vi "AlliGator Add Phasor Value to Plot v2.vi"(0 "Phasor Graph Ref":refnum<vi>, 1 "Calibration Phasor":T12, 5 "Phasor Data in":T2 {"[Phasor Graph:Raw Phasor Plots]"."[Decay Metadata]"."# Folds" min=1; "[Phasor Graph:Raw Phasor Plots]"."[Decay Metadata]"."ROI Descriptor"."Contours"."Type" items=["No Selection", "Point", "Line", "Rectangle", "Oval", "Polygon", "Freehand Region", "Annulus", "Unused2", "Unused3", "Broken Line", "Freehand Line", "Rotated Rectangle"]}, 7 "Decay":cluster{"t Array":dbl[], "I Array":dbl[]}, 9 "ROI Decay  Metadata":T4={"ROI Descriptor"={"Global Rectangle"=[], "Contours"=[]}, "ROI Center"={"X"=0, "Y"=0}, "Decay Background Subtraction Info"={"Laser Period"=0.0, "Gate Duration"=0.0, "Baseline Subtraction Method"=enum."Mean", "Background Definition Range"={"Min Gate"=0.0, "Max Gate"=0.0}, "Total Intensity w/o Bkgd Subtraction"=0.0, "Bkgd-subtracted Intensity (exp)"=0.0, "# Data Points"=0, "Background/Gate"=0.0, "Fitted Lifetime"=0.0, "Bkgd-subtracted Intensity (theo)"=0.0}, "Decay Reverted"=FALSE, "Decay Smoothened"=FALSE, "Decay Straightened"=FALSE, "Fitted Tau (Decay Straightening)"=0.0, "Decay Shift Parameters"={"Type"=enum."Default", "Shift"=0.0, "Threshold"=0.0, "Rotate"=FALSE}, "Decay Shifted"=FALSE, "Decay Extrapolated"=FALSE, "Decay Extrapolation Parameters"={"Additional Points"=0, "Head Fraction"=0.0, "Fitted Tau"=0.0, "Use Periodicity"=FALSE, "Use Cursors"=FALSE, "Tail Fraction"=0.0}, "Decay Normalized"=FALSE, "Fold Decay"=FALSE, "# Folds"=1} {"# Folds" min=1; "ROI Descriptor"."Contours"."Type" items=["No Selection", "Point", "Line", "Rectangle", "Oval", "Polygon", "Freehand Region", "Annulus", "Unused2", "Unused3", "Broken Line", "Freehand Line", "Rotated Rectangle"]}, 11 "Error In":errorcluster, 12 "Single Step Phasor":refnum<vi>) -> (2 "Raw Phasor":T1, 3 "Calibrated Phasor":T1, 4 "Phasor Data out":T2 {"[Phasor Graph:Raw Phasor Plots]"."[Decay Metadata]"."# Folds" min=1; "[Phasor Graph:Raw Phasor Plots]"."[Decay Metadata]"."ROI Descriptor"."Contours"."Type" items=["No Selection", "Point", "Line", "Rectangle", "Oval", "Polygon", "Freehand Region", "Annulus", "Unused2", "Unused3", "Broken Line", "Freehand Line", "Rotated Rectangle"]}, 8 "Raw Phasor SDV":T1, 10 "Calibrated Phasor SDV":T1, 13 "Apparent Phase Lifetime":dbl[unit], 14 "Message":string, 15 "Error Out":errorcluster)   [LabVIEW 2021, in "AlliGator Phasor Graph.lvlib"]
doc: "Core VI handling the creation of a phasor plot in the Phasor Graph.\n\nFrom the <B>Decay</B> plot and <B>Calibration Phasor</b>, computes the phasor (and if selected, the phasor standard deviation due to shot noise) and adds it to the current Phasor Plot in the Phasor Graph."
uses:
  AlliGator Phasor Graph.lvlib
  Phasor/Phasor (g, s).ctl
  Phasor/Calibration Phasor (m, phi).ctl
  AlliGator Decay Metadata v3.ctl
  Decay Analysis/Decay Preprocessing/AlliGator Decay Background Subtraction Info.ctl
  Decay Analysis/Decay Preprocessing/AlliGator Baseline Subtraction Method.ctl
  Graphs/XY Graph/XY Graph Plot Shift Parameters.ctl
  Graphs/XY Graph/XY Graph Plot Shift Method.ctl
  Decay Analysis/Decay Preprocessing/AlliGator Decay Extrapolation Parameters.ctl
  AlliGator Phasor Data.ctl
  AlliGator Raw Phasor Plot Data v4.ctl
  Phasor/Phasor Standard Deviation Options.ctl
  Settings/AlliGator Settings List.ctl
  Globals, Variables, Constants/AlliGator Variables List.ctl
  AlliGator Raw Phasor Plot Array Action.ctl
  dd0b4273-0e3d-468f-9a24-7a5fea4f6c4e.vi
  Variant/Variant to Data/Variant to Boolean.vi
  Phasor/Phasor.lvlib
  Settings/AlliGator Settings.lvlib
  Graphs/XY Graph/XY Graph Add-Ons.lvlib
  Error/Error.lvlib
  Phasor Ratio/AlliGator Phasor Ratio.lvlib
  Globals, Variables, Constants/AlliGator Globals, Variables & Constants.lvlib
  Variant/Variant to Data/Variant to Data.lvlib
  Decay Analysis/Decay Preprocessing/AlliGator Decay Preprocessing.lvlib
panel:
  # "see the AlliGator License on the block diagram (Ctrl+E or Window:Show Block Diagram)"
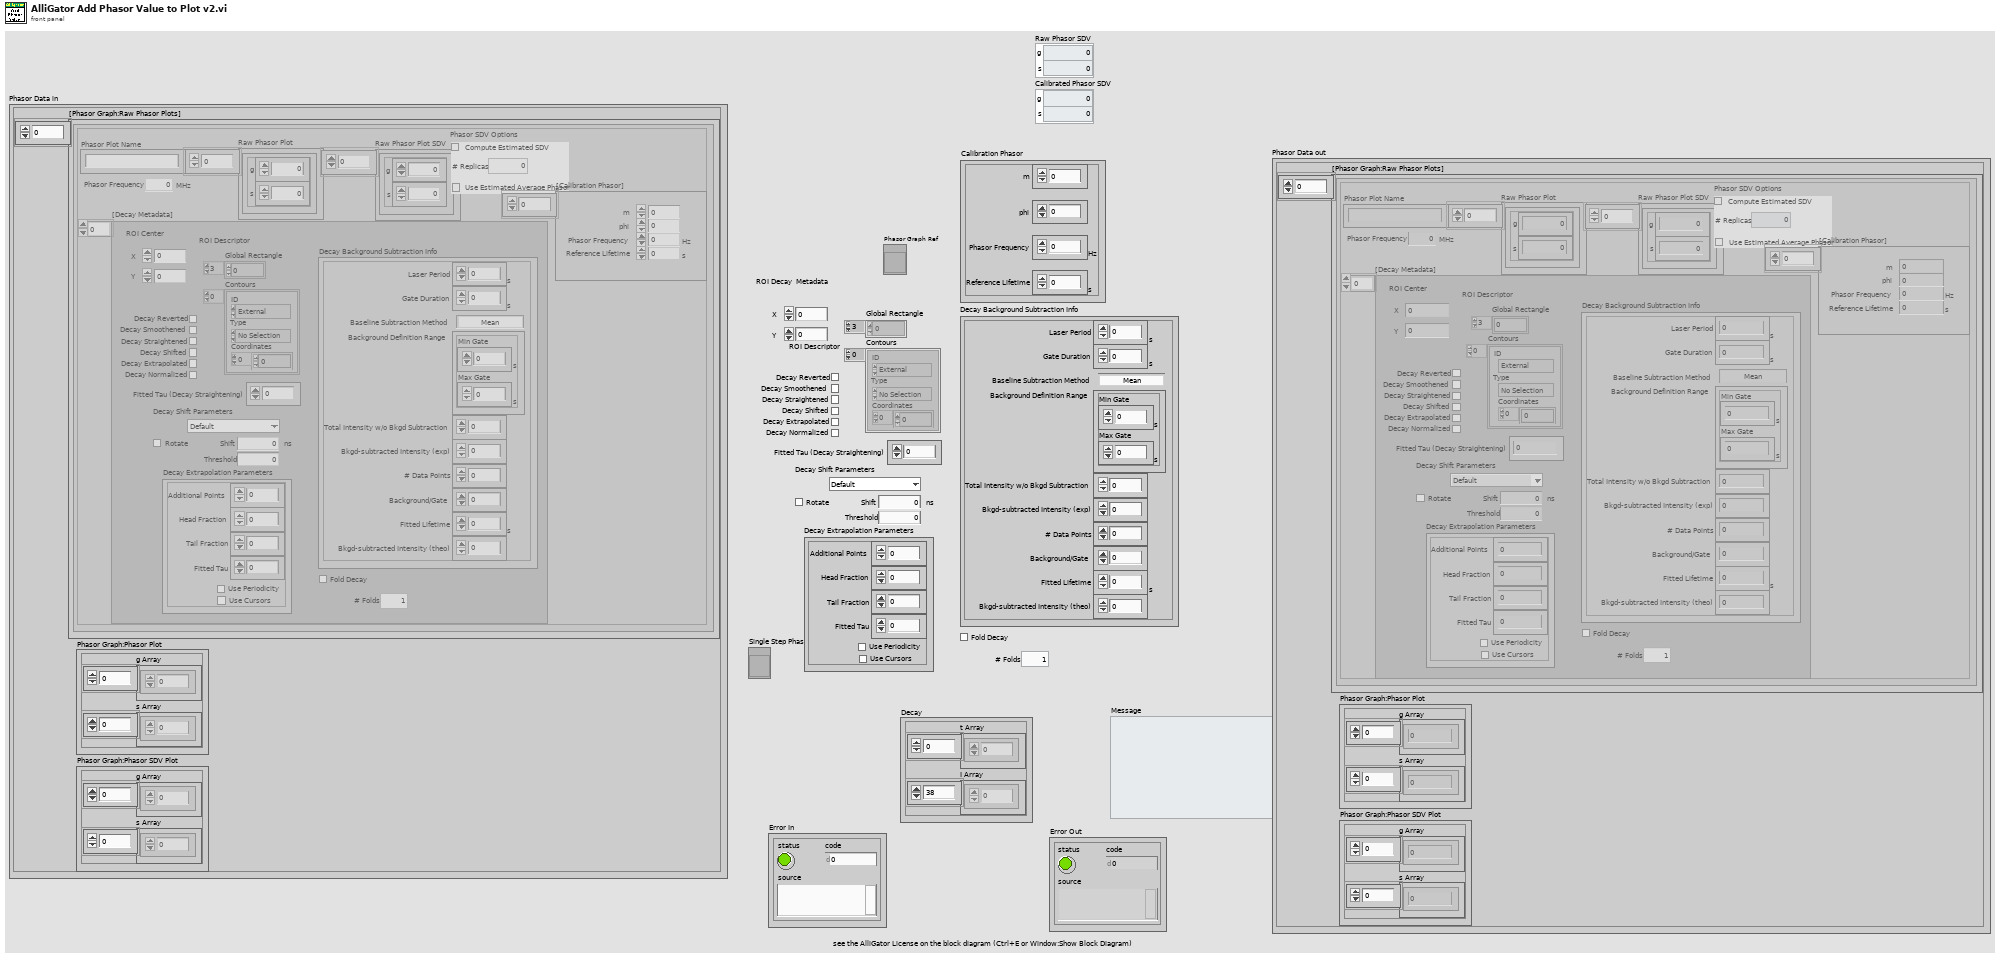
[diagram p1: front panel]
types:
  T1 = typedef "Phasor.lvlib/Phasor (g, s).ctl" = cluster{"g":dbl, "s":dbl}
  T2 = typedef "AlliGator Phasor Graph.lvlib/AlliGator Phasor Data.ctl" = cluster{"[Phasor Graph:Raw Phasor Plots]":T3[], "Phasor Graph:Phasor Plot":cluster{"g Array":dbl[], "s Array":dbl[]}, "Phasor Graph:Phasor SDV Plot":cluster{"g Array":dbl[], "s Array":dbl[]}}
  T3 = typedef "AlliGator Phasor Graph.lvlib/AlliGator Raw Phasor Plot Data v4.ctl" = cluster{"Phasor Plot Name":string, "Raw Phasor Plot":T1[], "Phasor Frequency":dbl[unit], "[Decay Metadata]":T4[], "Raw Phasor Plot SDV":T1[], "Phasor SDV Options":T11, "[Calibration Phasor]":T12[]}
  T4 = typedef "AlliGator Phasor Graph.lvlib/AlliGator Decay Metadata v3.ctl" = cluster{"ROI Descriptor":T5, "ROI Center":cluster{"X":i32, "Y":i32}, "Decay Background Subtraction Info":T6, "Decay Reverted":bool, "Decay Smoothened":bool, "Decay Straightened":bool, "Fitted Tau (Decay Straightening)":dbl, "Decay Shift Parameters":T8, "Decay Shifted":bool, "Decay Extrapolated":bool, "Decay Extrapolation Parameters":T10, "Decay Normalized":bool, "Fold Decay":bool, "# Folds":u32}
  T5 = typedef "ROI Descriptor" = cluster{"Global Rectangle":i32[], "Contours":cluster{"ID":enum32{"External", "Internal"}, "Type":u32, "Coordinates":i32[]}[]}
  T6 = typedef "AlliGator Decay Preprocessing.lvlib/AlliGator Decay Background Subtraction Info.ctl" = cluster{"Laser Period":dbl[unit], "Gate Duration":dbl[unit], "Baseline Subtraction Method":T7, "Background Definition Range":cluster{"Min Gate":dbl[unit], "Max Gate":dbl[unit]}, "Total Intensity w/o Bkgd Subtraction":dbl, "Bkgd-subtracted Intensity (exp)":dbl, "# Data Points":i32, "Background/Gate":dbl, "Fitted Lifetime":dbl[unit], "Bkgd-subtracted Intensity (theo)":dbl}
  T7 = typedef "AlliGator Decay Preprocessing.lvlib/AlliGator Baseline Subtraction Method.ctl" = enum16{"Mean", "Min", "Square Gated Single-Exponential", "File", "Constant"}
  T8 = typedef "XY Graph Add-Ons.lvlib/XY Graph Plot Shift Parameters.ctl" = cluster{"Type":T9, "Shift":dbl[unit], "Threshold":dbl, "Rotate":bool}
  T9 = typedef "XY Graph Add-Ons.lvlib/XY Graph Plot Shift Method.ctl" = enum16{"Default", "CFD", "Threshold", "Cross-Correlation"}
  T10 = typedef "AlliGator Decay Preprocessing.lvlib/AlliGator Decay Extrapolation Parameters.ctl" = cluster{"Additional Points":u32, "Head Fraction":dbl, "Fitted Tau":dbl, "Use Periodicity":bool, "Use Cursors":bool, "Tail Fraction":dbl}
  T11 = typedef "Phasor.lvlib/Phasor Standard Deviation Options.ctl" = cluster{"Compute Estimated SDV":bool, "# Replicas":u32, "Use Estimated Average Phasor":bool}
  T12 = typedef "Phasor.lvlib/Calibration Phasor (m, phi).ctl" = cluster{"m":dbl, "phi":dbl, "Phasor Frequency":dbl[unit], "Reference Lifetime":dbl[unit]}
  T13 = typedef "AlliGator Settings.lvlib/AlliGator Settings List.ctl" = enum16{"GUI:Visible Settings Tab", "GUI:Last Run Version", "Source Image:Use Image Histogram for Contrast", "Source Image:Low Count Pixels Rejection Options", "Source Image:High Count Pixels Rejection Options", "Source Image:Use Image Brightness", "Source Image:Blend Overlay with Image Background", "Source Image:Use Fixed ROI Diameter", "Source Image:ROI Diameter", "Source Image:ROI Center Color", "Source Image:Peak Threshold", "Source Image:Intensity Threshold", "Source Image:Image Binning Options", "Source Image:Image Smoothing Options", "Source Image:Image Histogram Active", "Source Image:Invert Binary Mask", "Source Image:Hot Pixel Removal", "Source Image:Overlay Analyzed ROI Center", "Source Image:Auto-Adjust Contrast", "Source Image:Histogram Lower Percentile", "Source Image:Histogram Upper Percentile", "Source Image:Save Source Image", "Source Image:Scale Bar Options", "Source Image:Image Resolution (Pixel Size)", "Source Image:Flatfield Correction", "Source Image:Show Dead Left Columns Correction", "Source Image:Dead Left Columns Correction", "Source Image:Image Pre-Processing Operations Order", "Source Image:Overlay ROI Median", "Source Image:Median Overlay Color", "Data Information:Gate Width", "Data Information:Nanotime Gate Separation", "Data Information:Macrotime Gate Separation", "Data Information:Gate Step", "Data Information:# Gates", "Data Information:Gate Image Exposure", "Data Information:Gate Image Integration", "Data Information:Gates to Skip", "Data Information:Gates to Keep", "Data Information:Define Gates to", "Data Information:Channel Name", "Data Information:Available Channel Names", "Data Information:Channel Arithmetic", "Data Information:Background File Subtraction", "Data Information:Background File", "Data Information:Background Scaling Factor", "Data Information:Background Pile-up Correction", "Data Information:Background Pixel Well Capacity", "Data Information:Laser Period", "Data Information:SYNC Period", "Data Information:Pile-up Correction", "Data Information:Pixel Well Capacity", "Data Information:Dataset Scaling Factor", "Fluorescence Decay_Decay Pre-Processing:Reverse Gates", "Fluorescence Decay_Decay Pre-Processing:Verbose Decay Pre-Processing", "Fluorescence Decay_Decay Pre-Processing:Use Decay Pre-Processing", "Fluorescence Decay_Decay Pre-Processing:Background Subtraction", "Fluorescence Decay_Decay Pre-Processing:Background Definition Range", "Fluorescence Decay_Decay Pre-Processing:Baseline Subtraction Method", "Fluorescence Decay_Decay Pre-Processing:Decay Pre-Processing Operations Order", "Fluorescence Decay_Decay Pre-Processing:Smoothing Parameter", "Fluorescence Decay_Decay Pre-Processing:Shift Decay", "Fluorescence Decay_Decay Pre-Processing:Decay Shift Parameters", "Fluorescence Decay_Decay Pre-Processing:Fold Decay", "Fluorescence Decay_Decay Pre-Processing:# Folds", "Fluorescence Decay_Decay Pre-Processing:1-Normalize Decay", "Fluorescence Decay_Decay Pre-Processing:[0-1]-Normalize Decay", "Fluorescence Decay_Decay Pre-Processing:Smoothen Decay", "Fluorescence Decay_Decay Pre-Processing:Extrapolate Decay", "Fluorescence Decay_Decay Pre-Processing:Use Periodicity", "Fluorescence Decay_Decay Pre-Processing:Use Cursors", "Fluorescence Decay_Decay Pre-Processing:Tail Fraction", "Fluorescence Decay_Decay Pre-Processing:Head Fraction", "Fluorescence Decay_Decay Pre-Processing:Additional Points", "Fluorescence Decay_Decay Pre-Processing:Straighten Decay", "Fluorescence Decay_Decay Pre-Processing:Constant Background", "Fluorescence Decay_Decay Pre-Processing:Pixel-Normalize Decay", "Fluorescence Decay_Advanced Analysis:Extract IRF instead of Decay", "Fluorescence Decay_Advanced Analysis:IRF Extraction Options", "Fluorescence Decay_Advanced Analysis:IRF Optimization Options", "Fluorescence Decay_Advanced Analysis:Square Pulse Options", "Fluorescence Decay_Advanced Analysis:IRF Order", "Fluorescence Decay_Advanced Analysis:IRF Time Constants", "Fluorescence Decay_Advanced Analysis:Wavelet Analysis Options", "Fluorescence Decay_Advanced Analysis:Average Lifetime Options", "Fluorescence Decay_Fit Options:Fit Options", "Fluorescence Decay_Fit Options:Use Legacy Fitting Approach", "Fluorescence Decay_Fit Options:Use Data Information Laser Period", "Fluorescence Decay_Fit Parameters:Displayed Fit Parameters", "Fluorescence Decay_Fit Parameters:Fit Parameter Constraints", "Fluorescence Decay_Fit Parameters:Export Tabulated Results", "Fluorescence Decay_Fit Parameters:MLE Baseline Offset Type", "Fluorescence Decay_Fit Parameters:MLE Baseline Offset", "Fluorescence Decay_Fit Parameters:Guess Parameter Names", "Fluorescence Decay_Fit Parameters:Guess Parameter Values", "Fluorescence Decay_Fit Parameters:Guess Parameters Options", "Fluorescence Decay_Styles:Show Last Decay Only", "Fluorescence Decay_Styles:Decay Graph Color Array", "Fluorescence Decay:Decay Graph Active", "Fluorescence Decay Statistics:Min Peak Value", "Fluorescence Decay Statistics:Reject Low Decay Peak Pixels", "Fluorescence Decay Statistics:Reject High Decay Peak Pixels", "Fluorescence Decay Statistics:Max Peak Value", "Time Traces:Use File Timestamp", "Time Traces:Time Step", "Time Traces:Use Intensity Correction File", "Time Traces:Intensity Correction File", "Phasor Plot:Phasor Plot Smoothing Options", "Phasor Plot:Phasor Plot Size", "Phasor Plot:Phasor Plot Graphics Options", "Phasor Plot:Cumulative Phasor Plot", "Phasor Plot:Use Phasor Brightness", "Phasor Plot:Blend Overlay with Phasor Background", "Phasor Plot:Save Phasor Plot", "Phasor Plot:Show References", "Phasor Plot:Phasor Ratio Decay Range", "Phasor Plot:Exponential Fading", "Phasor Plot:Phasor Ratio Reference Colors", "Phasor Plot:Reference Radius", "Phasor Plot:Show Color Map Vertices", "Phasor Plot:Phasor Plot Active", "Phasor Plot:Phasor Ratio Color Map Type", "Phasor Plot:Phasor Ratio Color Map", "Phasor Plot:Phasor Ratio Display Range", "Phasor Plot:Selected Image ROI(s)", "Phasor Plot:All Image ROIs", "Phasor Plot:Selected Phasor Plot ROI(s)", "Phasor Plot:All Phasor Plot ROIs", "Phasor Plot:Phasor Ratio Color-Coded Quantity", "Phasor Plot:Store Phasor Harmonics", "Phasor Plot:Draw Reference Segment", "Phasor Plot:User-Defined Quantity", "Phasor Graph:Phasor Frequency", "Phasor Graph:Phasor Ratio Type", "Phasor Graph:Pixel-level Phasor Computation", "Phasor Graph:Save Phasor Graph", "Phasor Graph:Phasor Graph Active", "Phasor Graph:Phasor SDV Options", "Phasor Calibration:Use Backup Calibration if needed", "Phasor Graph:Define Shortest Lifetime as", "Phasor Calibration:Backup Calibration Type", "Phasor Calibration:Calibration Type", "Phasor Calibration:Calibration Lifetime", "Phasor Calibration:Calibration Map Algorithm", "Single-Exponential Phasor Locus (SEPL):Gate Parameters", "Single-Exponential Phasor Locus (SEPL):User-defined Gate", "Single-Exponential Phasor Locus (SEPL):User-defined IRF", "Single-Exponential Phasor Locus (SEPL):Phasor Parameters", "Single-Exponential Phasor Locus (SEPL):Decay & IRF Parameters", "Single-Exponential Phasor Locus (SEPL):Display Parameters", "Lifetime Analysis:Decay Analysis Parameters", "Lifetime Analysis:Lifetime Map Active", "Plugins:Python Settings", "Miscellaneous:Verbose Mode", "Miscellaneous:Beep after Script", "Miscellaneous:Saved Image File Format", "Miscellaneous:Exported Gate Image Settings", "Miscellaneous:Include Loading in Timing", "Miscellaneous:Verbose Settings Mode", "Miscellaneous:Histogram Options", "Miscellaneous:Beep on Error", "Miscellaneous:# Logical Processors Used", "Miscellaneous:ROI Description Max Characters", "Miscellaneous:Verbose Error Mode", "Miscellaneous:Transparent Mask Color"}
  T14 = typedef "AlliGator Globals, Variables & Constants.lvlib/AlliGator Variables List.ctl" = enum16{"---- GUI ----", "GUI:Initialization Status", "GUI:State Indicators Refnum", "GUI:Original AlliGator Menu Items", "GUI:Current Action Loop State", "GUI:Script in progress", "GUI:Playback", "GUI:Loop Playback", "GUI:Search ROI Used", "GUI:Search ROI", "Decay Graph Max Legend Size", "Intensity Graph Max Legend Size", "Decay Statistics Graph Max Legend Size", "Phasor Graph Max Legend Size", "Phasor Ratio Graph Max Legend Size", "Lifetime Graph Max Legend Size", "---- Files ----", "Files:Export Dataset Frames as Individual Files", "Files:Show Batch Export Help Balloons", "Files:Frames in Dataset", "Files:ptu File Frame Start Indices", "Files:Current Frame in Dataset", "Files:Current Frame Timestamp", "Files:Dataset Loaded", "Files:Dataset Metadata", "Files:Dataset Channel", "Files:Dataset Data Description", "Files:Background Dataset Metadata", "Files:Background Dataset Channel", "Files:Background Dataset Data Description", "Files:Background File Subtraction", "Files:Background File Path", "Files:Background File Pile-up Correction", "Files:Background File Pixel Well Capacity", "Files:Background File Scaling Factor", "Files:Current Dataset Load Settings", "Files:Dataset Path", "Files:ICCD-specific Information", "Files:Macrotime Gate Separation", "------ Python Plugins ------", "Python Plugins:Information", "Python Plugins:Python Session", "Python Plugins:Valid Python Session?", "---- Source Image ----", "Source Image:ROIs", "Source Image:Current ROI", "Source Image:ROI Event Refnum", "X_Source Image Display Range", "X_Source Image Palette Information", "X_Type of Displayed Image", "X_Time Gate Slider", "Source Image:Palette List", "Source Image:Scale", "Source Image:ROI Overlay Color", "Source Image:Overlay to Erase", "Source Image:Is Displayed Image Accumulated", "Source Image:White Light Image Modified", "Source Image:Mask Image Modified", "---- Image Profile Window ----", "Image Profile:Window Event Refnum", "Image Profile:IntensityType", "Image Profile:Intensity Average Type", "Image Profile:Intensity-weighted SDV", "Image Profile:Box Profile Type", "Image Profile:Window Open", "Image Profile:Plotted Fit Parameter", "------ Phasor Graph -------", "Phasor Graph:Show Line", "---- Phasor Plot ---", "Phasor Plot:Parameters Changed", "Phasor Plot:FLI Dataset Modified since last Calculation", "Phasor Harmonics Data", "Selected Phasor Harmonics", "Phasor Harmonic Manager Event Refnum", "Phasor Plot:ROIs", "Phasor Plot:Current ROI", "Phasor Plot:ROI Event Refnum", "Phasor Plot:Image Reference Points", "Phasor Plot:Computed", "Phasor Plot:Palette Information", "Phasor Plot:Palette List", "Phasor Plot:Phasor Ratio Palette Information", "Phasor Plot:Phasor Ratio Palette List", "Phasor Plot:Image Scale", "Phasor Plot:Image Overlay to Erase", "Phasor Plot:Image Elements to Update", "Phasor Plot:Current Calculation Parameters", "Phasor Plot:Current Calibration Options", "Phasor Plot:Reset Cumulated Phasor Plot", "Phasor Plot:Reference 1", "Phasor Plot:Lifetime Reference 1", "Phasor Plot:Reference 1 Frequency", "Phasor Plot:Reference 2", "Phasor Plot:Lifetime Reference 2", "Phasor Plot:Reference 2 Frequency", "---- Decay Analysis ----", "Number of Selected Decays to Fit", "LS Fit Results", "LAR Fit Results", "BS Fit Results", "Last Decay Max - Min", "Best Fit Parameters", "Best Fit Parameter Names", "Actual Size X", "Actual Size Y", "Binning X", "Binning Y", "Actual # Gates", "Dataset Number", "Gates to...", "Gates Skipped", "Gates to keep", "Gate Step", "Gate Separation", "Reversed Gates", "Pile-up Correction", "Pixel Well Capacity", "Background Subtracted", "Background Subtraction Method", "Background Definition Range", "Background File (deprecated)", "Number of Dataset Accumulated", "Array of Accumulated Dataset Paths", "Do Averaged Datasets", "Destination File Path", "Process Plot Target", "Use 1/D as Phasor Frequency", "---- Decay Fit Parameter Map -----", "Decay Fit Parameter Map:Palette Information", "Decay Fit Parameter Map:Palette List", "---- Parameter Map ----", "Parameter Map:Palette Information", "Parameter Map:Palette List", "------- Local Decay Window ---------", "Local Decay Graph Window:Event Refnum", "Local Decay Graph Window:Use normalized IRF for convolution", "----- Miscellaneous ----", "Misc:Skippable Dialog Windows Status"}
  T15 = typedef "AlliGator Phasor Graph.lvlib/AlliGator Raw Phasor Plot Array Action.ctl" = enum16{"Clear All", "-", "Add Raw Phasor Plot", "Delete Raw Phasor Plot", "Replace Raw Phasor Plot", "---------------------", "Add Phasor to Plot", "Replace Phasor in Plot", "Remove Phasor in Plot"}
  T16 = typedef "XY Graph Add-Ons.lvlib/XY Graph Refnum.ctl" = refnum<vi>
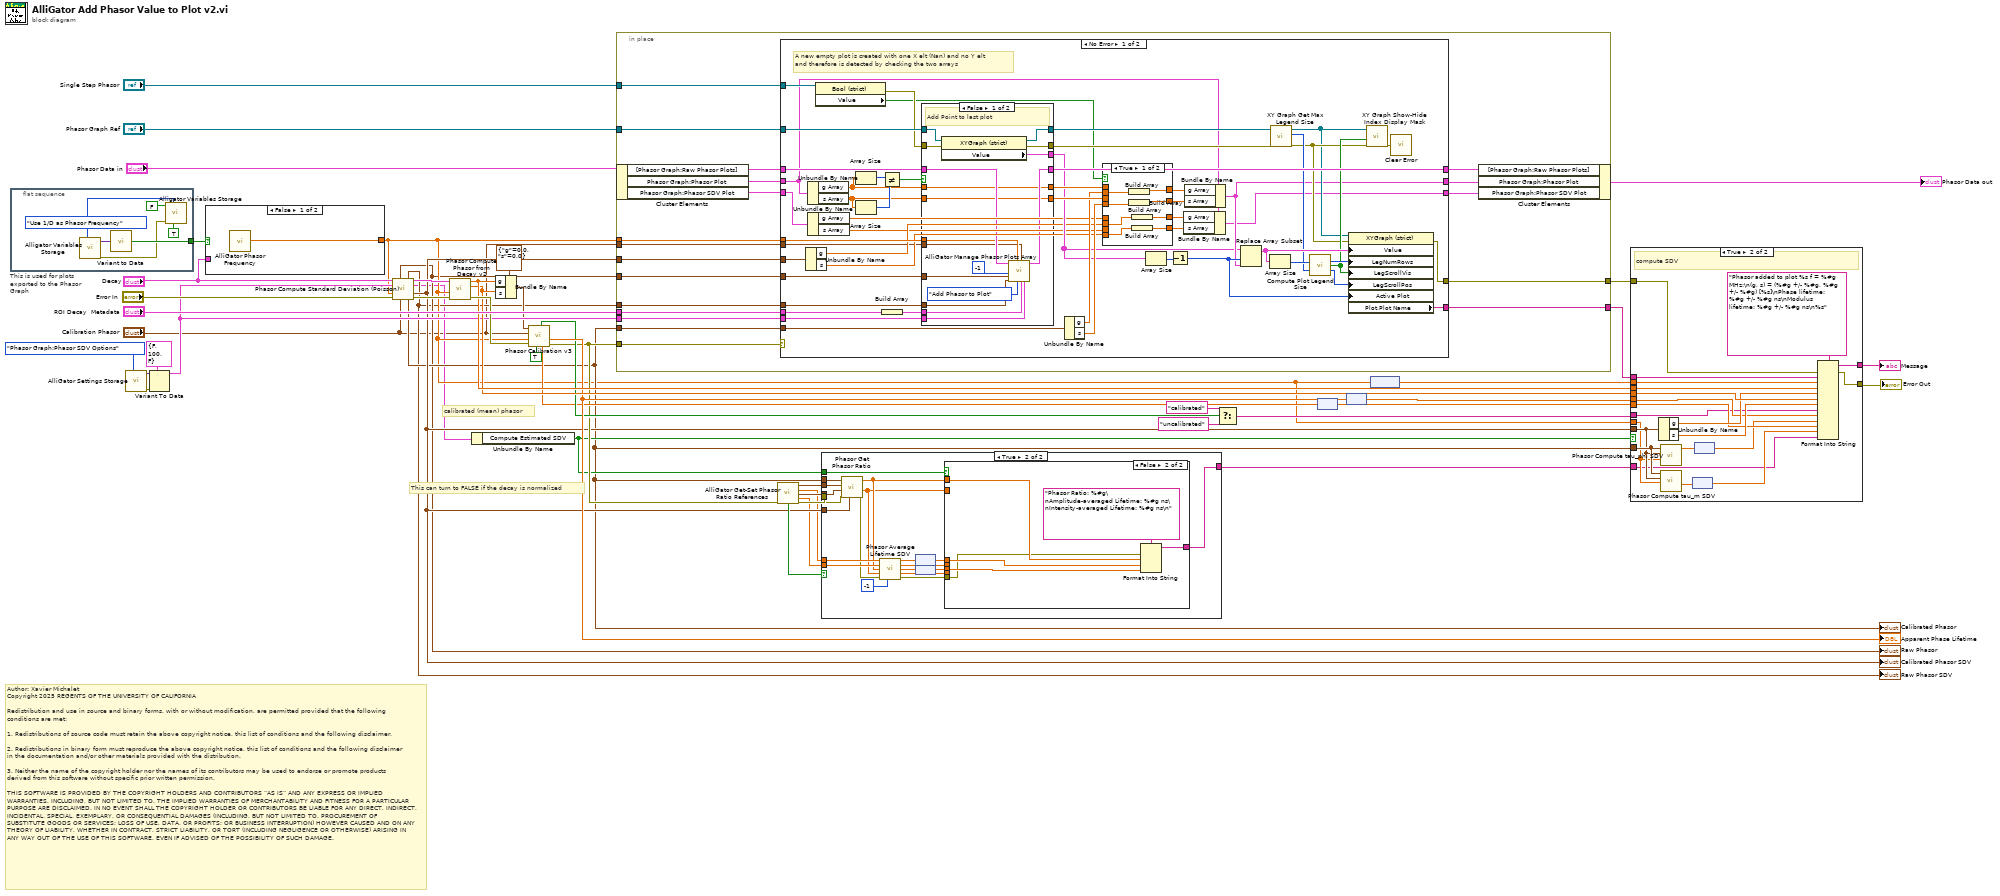
[diagram p0: block diagram]
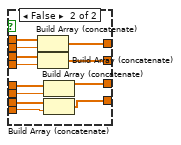
[diagram p2: hidden frame]
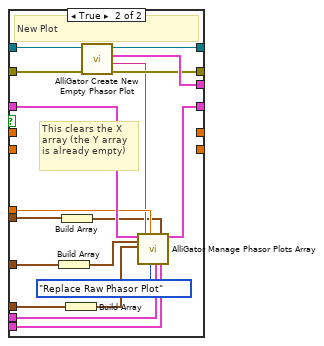
[diagram p3: hidden frame]
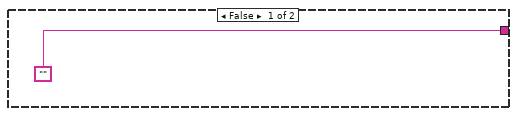
[diagram p5: hidden frame]
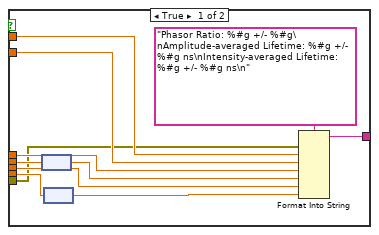
[diagram p6: hidden frame]
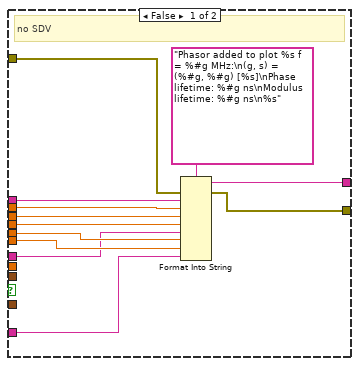
[diagram p7: hidden frame]
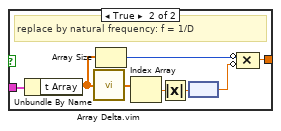
[diagram p8: hidden frame]
diagram:
  # "Author: Xavier Michalet\nCopyright 2025 REGENTS OF THE UNIVERSITY OF CALIFORNIA\n\nRedistribution and use in source and binary forms, with or without modification, are permitted provided that the following conditions are met:\n\n1. Redistributions of source code must retain the above copyright notice, this list of conditions and the following disclaimer.\n\n2. Redistributions in binary form must reproduce the above copyright notice, this list of conditions and the following disclaimer in the documentation and/or other materials provided with the distribution.\n\n3. Neither the name of the copyright holder nor the names of its contributors may be used to endorse or promote products derived from this software without specific prior written permission.\n\nTHIS SOFTWARE IS PROVIDED BY THE COPYRIGHT HOLDERS AND CONTRIBUTORS “AS IS” AND ANY EXPRESS OR IMPLIED WARRANTIES, INCLUDING, BUT NOT LIMITED TO, THE IMPLIED WARRANTIES OF MERCHANTABILITY AND FITNESS FOR A PARTICULAR PURPOSE ARE DISCLAIMED. IN NO EVENT SHALL THE COPYRIGHT HOLDER OR CONTRIBUTORS BE LIABLE FOR ANY DIRECT, INDIRECT, INCIDENTAL, SPECIAL, EXEMPLARY, OR CONSEQUENTIAL DAMAGES (INCLUDING, BUT NOT LIMITED TO, PROCUREMENT OF SUBSTITUTE GOODS OR SERVICES; LOSS OF USE, DATA, OR PROFITS; OR BUSINESS INTERRUPTION) HOWEVER CAUSED AND ON ANY THEORY OF LIABILITY, WHETHER IN CONTRACT, STRICT LIABILITY, OR TORT (INCLUDING NEGLIGENCE OR OTHERWISE) ARISING IN ANY WAY OUT OF THE USE OF THIS SOFTWARE, EVEN IF ADVISED OF THE POSSIBILITY OF SUCH DAMAGE."
  # "This can turn to FALSE if the decay is normalized"
  # "calibrated (mean) phasor"
  n1 = flat-sequence "This is used for plots exported to the Phasor Graph" {
    tunnel: [w55] -> w8
    frame #0 {
      w53 = AlliGator_Variables_List."Use 1/D as Phasor Frequency" ("AlliGator Variable")
      n2 = call "Alligator Variables Storage.vi"("AlliGator Variable"=w53) -> ("Error Out"=w54:errorcluster, "Data out"=w56:variant)  [unwired: 8 in, 1 out]
      n3 = call-poly "Variant to Data.vi"("Variant"=w56) -> ("Value"=w55:bool)  [unwired: 8 in]
      n4 = call "Alligator Variables Storage.vi"("Get(F)/Set"=TRUE, "AlliGator Variable"=w53, "Error In"=w54, "Data in"=FALSE ("Value")) -> ()  [unwired: 5 in, 3 out]
    }
  }
  n5 = call "AlliGator Settings Storage.vi"("AlliGator Settings List"=AlliGator_Settings_List."Phasor Graph:Phasor SDV Options") -> ("Error Out"=w35:errorcluster, "Variant Data out"=w34:variant)  [unwired: 9 in]
  n6 = Variant To Data(error in=w35, type=T11 {"Compute Estimated SDV"=FALSE, "# Replicas"=100, "Use Estimated Average Phasor"=FALSE} ("Phasor SDV Options"), Variant=w34) -> (data=w24:T11)  [unwired: 1 out]
  n7 = case shown="False" w8 {
    tunnel: [w57 w60] -> w7
    tunnel: "Decay" -> [_ w65]
    frame False {
      n8 = call "AlliGator Phasor Frequency.vi"() -> ("Phasor Frequency"=w57:dbl[unit])
    }
    frame True {
      # "replace by natural frequency: f = 1/D"
      n9 = Unbundle By Name(w65) -> ("t Array"=w64:dbl[])
      n10 = call "Array Delta.vim"("A"=w64) -> ("A[i+1]-A[i]"=w63:dbl[])  [unwired: 8 in]
      n11 = Array Size(array=w64) -> (size(s)=w62:i32)
      n12 = Index Array(array=w63) -> (element=w61:dbl)  [unwired: 1 in]
      n13 = Absolute Value(x=w61) -> (abs(x)=w58:dbl)
      n14 = node(w58) -> (w59:dbl[unit])
      n15 = Compound Arithmetic op=MULTIPLY(invert w62, invert w59) -> (w60:dbl[unit])
    }
  }
  n16 = call "Phasor Compute Standard Deviation (Poisson).vi"("Time-Gated Decay"="Decay", "Phasor SDV Options in"=w24, "Phasor Frequency"=w7, "Error In"="Error In", "Calibration Phasor (m, phi)"="Calibration Phasor") -> ("(Mean) Phasor (g, s)"=w6:T1, "Phasor SDV (g, s)"=w5:T1, "Time-Gated Decay (dup)"=w28:cluster{"t Array":dbl[], "I Array":dbl[]}, "Phasor SDV Options out"=w4:T11, "Calibrated Phasor SDV (g, s)"=w14:T1, "Calibrated (Mean) Phasor (g, s)"=w9:T1, "Error Out"=w29:errorcluster)  [unwired: 4 in]
  "Calibrated Phasor" <- w9
  "Raw Phasor" <- w6
  "Raw Phasor SDV" <- w5
  "Calibrated Phasor SDV" <- w14
  n17 = call "Phasor Compute Phasor from Decay v2.vi"("Error In"=w29, "Phasor Frequency"=w7, "Time-Gated Decay"=w28) -> ("Error Out"=w46:errorcluster, "s"=w40:dbl, "g"=w41:dbl)  [unwired: 5 in, 1 out]
  n18 = Unbundle By Name(w4) -> ("Compute Estimated SDV"=w13:bool)
  n19 = Bundle By Name(cluster=T1 {"g"=0.0, "s"=0.0} ("Phasor"), "g"=w41, "s"=w40) -> (w10:T1)
  n20 = call "Phasor Calibration v3.vi"("Compute Lifetimes? (F)"=TRUE ("Init?"), "Error In"=w46, "Phasor Frequency"=w7, "Calibration Phasor"="Calibration Phasor", "Measured Phasor"=w10) -> ("Error Out"=w17:errorcluster, "Calibrated Phase Lifetime"=w39:dbl[unit], "Calibrated Modulus Lifetime"=w26:dbl[unit], "Calibrated?"=w27:bool)  [unwired: 1 in, 2 out]
  "Apparent Phase Lifetime" <- w39
  n21 = in-place {
    in-place-border: "Phasor Graph Ref" -> [w84]
    in-place-border: "Single Step Phasor" -> [w83]
    in-place-border: "ROI Decay  Metadata" -> [w82]
    in-place-border: [w81] -> w44
    in-place-border: [w80] -> w43
    in-place-border: w24 -> [w79]
    in-place-border: w17 -> [w78]
    in-place-border: w14 -> [w77]
    in-place-border: w9 -> [w76]
    in-place-border: w7 -> [w75]
    in-place-border: w6 -> [w74]
    in-place-border: w5 -> [w73]
    in-place-border: "Calibration Phasor" -> [w72]
    n22 = in-place-cluster #1("Phasor Data in") -> ("[Phasor Graph:Raw Phasor Plots]"=w71:T3[], "Phasor Graph:Phasor Plot"=w70:cluster{"g Array":dbl[], "s Array":dbl[]}, "Phasor Graph:Phasor SDV Plot"=w69:cluster{"g Array":dbl[], "s Array":dbl[]})
    n23 = case shown="No Error" w78 {
      selector: w78 -> [_ w193]
      tunnel: w84 -> [w136 _]
      tunnel: w76 -> [w135 _]
      tunnel: [w104 w194] -> w67
      tunnel: w83 -> [w134 _]
      tunnel: w70 -> [w95 w194]
      tunnel: w74 -> [w131 _]
      tunnel: w71 -> [w130 w195]
      tunnel: [w129 w195] -> w68
      tunnel: w75 -> [w126 _]
      tunnel: w82 -> [w124 _]
      tunnel: [w102 w193] -> w81
      tunnel: [w103 _] -> w80
      tunnel: w73 -> [w98 _]
      tunnel: w79 -> [w97 _]
      tunnel: w69 -> [w88 w192]
      tunnel: [w94 w192] -> w66
      tunnel: w77 -> [w93 _]
      tunnel: w72 -> [w85 _]
      frame No Error {
        # "A new empty plot is created with one X elt (Nan) and no Y elt\nand therefore is detected by checking the two arrays"
        n24 = Unbundle By Name(w93) -> ("g"=w92:dbl, "s"=w91:dbl)
        n25 = Unbundle By Name(w95) -> ("g Array"=w107:dbl[], "s Array"=w106:dbl[])
        n26 = Unbundle By Name(w88) -> ("g Array"=w87:dbl[], "s Array"=w86:dbl[])
        n27 = property class="Bool (strict)"(reference=w134) -> (error out=w113:errorcluster, "Value"=w96:bool)  [unwired: 1 in, 1 out]
        n28 = Array Size(array=w107) -> (size(s)=w112:i32)
        n29 = Array Size(array=w106) -> (size(s)=w111:i32)
        n30 = Not Equal?(x=w112, y=w111) -> (x != y?=w110:bool)
        n31 = Build Array(w124) -> (w125:T4[])
        n32 = case shown="False" w110 {
          tunnel: [w169 w191] -> w99
          tunnel: w136 -> [w173 w190]
          tunnel: w113 -> [w171 w189]
          tunnel: [w170 w188] -> w122
          tunnel: [w172 w187] -> w123
          tunnel: w131 -> [w165 w184]
          tunnel: w130 -> [w167 w186]
          tunnel: [w168 w185] -> w129
          tunnel: w126 -> [w161 w181]
          tunnel: w107 -> [w163 _]
          tunnel: w106 -> [w162 _]
          tunnel: [w163 _] -> w128
          tunnel: [w162 _] -> w127
          tunnel: w125 -> [w160 w179]
          tunnel: w98 -> [w159 w178]
          tunnel: w97 -> [w158 w176]
          tunnel: w85 -> [w157 w174]
          frame False {
            # "Add Point to last plot"
            n33 = property class="XYGraph (strict)"(reference=w173, error in=w171) -> (reference out=w172:refnum<vi>, error out=w170:errorcluster, "Value"=w169:cluster{"X Array":dbl[], "Y Array":dbl[]}[])
            n34 = call "AlliGator Manage Phasor Plots Array.vi"("[Raw Phasor Plot] in"=w167, "Plot Index (-1: Last)"=-1 ("Plot Index"), "Raw Phasor (g, s)"=w165, "Raw Phasor SDV"=w159, "Phasor Frequency"=w161, "[Raw Phasor Plot] Action"=AlliGator_Raw_Phasor_Plot_Array_Action."Add Phasor to Plot", "Calibration Phasor"=w157, "Phasor Metadata"=w160, "Phasor SDV Options"=w158) -> ("[Raw Phasor Plot] out"=w168:T3[])  [unwired: 10 in]
          }
          frame True {
            # "This clears the X array (the Y array is already empty)"
            # "New Plot"
            n35 = Build Array(w184) -> (w183:T1[])
            n36 = Build Array(w174) -> (w175:T12[])
            n37 = Build Array(w178) -> (w177:T1[])
            n38 = call "AlliGator Create New Empty Phasor Plot.vi"("Error In"=w189, "Phasor Graph Ref"=w190) -> ("Error Out"=w188:errorcluster, "Plot Name"=w180:string, "Plot Array out"=w191:cluster{"X Array":dbl[], "Y Array":dbl[]}[], "Phasor Graph Ref (dup)"=w187:refnum<vi>)  [unwired: 6 in]
            n39 = call "AlliGator Manage Phasor Plots Array.vi"("[Raw Phasor Plot] in"=w186, "Raw Phasor Plot (empty)"=w183, "Raw Phasor SDV Plot (empty)"=w177, "Plot Name"=w180, "Phasor Frequency"=w181, "[Raw Phasor Plot] Action"=AlliGator_Raw_Phasor_Plot_Array_Action."Replace Raw Phasor Plot", "Phasor Metadata"=w179, "[Calibration Phasor]"=w175, "Phasor SDV Options"=w176) -> ("[Raw Phasor Plot] out"=w185:T3[])  [unwired: 10 in]
          }
        }
        n40 = Unbundle By Name(w135) -> ("g"=w101:dbl, "s"=w100:dbl)
        n41 = case shown="True" w96 {
          tunnel: w101 -> [w144 w156]
          tunnel: w100 -> [w143 w155]
          tunnel: w128 -> [_ w154]
          tunnel: w127 -> [_ w153]
          tunnel: [w142 w152] -> w109
          tunnel: [w141 w151] -> w108
          tunnel: w92 -> [w140 w148]
          tunnel: w91 -> [w139 w146]
          tunnel: [w138 w149] -> w90
          tunnel: [w137 w145] -> w89
          tunnel: w87 -> [_ w150]
          tunnel: w86 -> [_ w147]
          frame True {
            n42 = Build Array(w144) -> (w142:dbl[])
            n43 = Build Array(w143) -> (w141:dbl[])
            n44 = Build Array(w140) -> (w138:dbl[])
            n45 = Build Array(w139) -> (w137:dbl[])
          }
          frame False {
            n46 = Build Array (concatenate)(w154, w156) -> (w152:dbl[])
            n47 = Build Array (concatenate)(w153, w155) -> (w151:dbl[])
            n48 = Build Array (concatenate)(w150, w148) -> (w149:dbl[])
            n49 = Build Array (concatenate)(w147, w146) -> (w145:dbl[])
          }
        }
        n50 = Array Size(array=w99) -> (size(s)=w132:i32)
        n51 = Decrement(x=w132) -> (x-1=w105:i32)
        n52 = Bundle By Name(cluster=w95, "g Array"=w90, "s Array"=w89) -> (w94:cluster{"g Array":dbl[], "s Array":dbl[]})
        n53 = Bundle By Name(cluster=w95, "g Array"=w109, "s Array"=w108) -> (w104:cluster{"g Array":dbl[], "s Array":dbl[]})
        n54 = Replace Array Subset(array=w99, new element=w104, index=w105) -> (w133:cluster{"X Array":dbl[], "Y Array":dbl[]}[])
        n55 = Array Size(array=w133) -> (size(s)=w121:i32)
        n56 = call "XY Graph Get Max Legend Size.vi"("Error In"=w122, "XYGraph Refnum"=w123) -> ("Error Out"=w116:errorcluster, "Max Legend Size"=w120:i32, "XYGraph Refnum"=w115:T16)  [unwired: 6 in, 1 out]
        n57 = call "Compute Plot Legend Size.vi"("# Plots"=w121, "Max Legend Size"=w120) -> ("LegNumRows"=w119:u32, "LegScrollVis"=w117:bool, "LegScrollPos"=w118:u32)  [unwired: 11 in]
        n58 = property class="XYGraph (strict)"(reference=w115, error in=w116, "Value"=w133, "LegNumRows"=w119, "LegScrollVis"=w117, "LegScrollPos"=w118, "Active Plot"=w105) -> (error out=w102:errorcluster, "Plot.Plot Name"=w103:string)  [unwired: 1 out]
        n59 = call "XY Graph Show-Hide Index Display Mask.vi"("error in (no error)"=w116, "Show(T)/Hide(F)"=w117, "XYGraph Ref"=w115) -> ("error out"=w114:errorcluster)  [unwired: 7 in, 1 out]
        n60 = call "Clear Error.vi"("Error In"=w114) -> ()  [unwired: 8 in, 1 out]
      }
      frame Error {
      }
    }
    n61 = in-place-cluster #1("[Phasor Graph:Raw Phasor Plots]"=w68, "Phasor Graph:Phasor Plot"=w67, "Phasor Graph:Phasor SDV Plot"=w66) -> (→"Phasor Data out":T2)
  }
  n62 = call "AlliGator Get-Set Phasor Ratio References.vi"("error in (no error)"=w17) -> ("All defined?"=w16:bool, "Reference Phasor 1"=w20:T1, "Reference Lifetime 1"=w12:dbl[unit], "Reference Phasor 2"=w19:T1, "Reference Lifetime 2"=w11:dbl[unit], "error out"=w18:errorcluster)  [unwired: 7 in, 2 out]
  n63 = case shown="True" w16 {
    tunnel: w20 -> [_ w216]
    tunnel: w19 -> [_ w215]
    tunnel: w9 -> [_ w214]
    tunnel: w18 -> [_ w213]
    tunnel: ["" w211] -> w15
    tunnel: w14 -> [_ w212]
    tunnel: w13 -> [_ w210]
    tunnel: w12 -> [_ w209]
    tunnel: w11 -> [_ w208]
    frame False {
    }
    frame True {
      n64 = call "Phasor Get Phasor Ratio.vi"("Phasor SDV"=w212, "Error In"=w213, "Reference Phasor 2"=w215, "Reference Phasor 1"=w216, "Phasor"=w214) -> ("Error Out"=w207:errorcluster, "Phasor Ratio SDV"=w205:dbl, "Phasor Ratio (f1)"=w206:dbl)  [unwired: 4 in]
      n65 = call "Phasor Average Lifetime SDV.vi"("tau 1"=w209, "tau 2"=w208, "r"=w206, "SDV r"=w205, "Error In"=w207, "seed"=-1) -> ("<tau>_a"=w204:dbl[unit], "SDV <tau>_a"=w203:dbl[unit], "<tau>_i"=w202:dbl[unit], "SDV <tau>_i"=w201:dbl[unit], "Error Out"=w200:errorcluster)  [unwired: 4 in, 1 out]
      n66 = node(w204) -> (w199:dbl)
      n67 = node(w202) -> (w198:dbl)
      n68 = case shown="False" w210 {
        tunnel: [w227 w233] -> w211
        tunnel: w206 -> [w226 w232]
        tunnel: w205 -> [w224 _]
        tunnel: w199 -> [w223 w230]
        tunnel: w203 -> [w222 _]
        tunnel: w198 -> [w221 w229]
        tunnel: w201 -> [w220 _]
        tunnel: w200 -> [w219 w228]
        frame True {
          n69 = node(w222) -> (w218:dbl)
          n70 = node(w220) -> (w217:dbl)
          n71 = Format Into String(format string="Phasor Ratio: %#g +/- %#g\nAmplitude-averaged Lifetime: %#g +/- %#g ns\nIntensity-averaged Lifetime: %#g +/- %#g ns\n", error in=w219, w226, w224, w223, w218, w221, w217) -> (resulting string=w227:string)  [unwired: 1 in, 1 out]
        }
        frame False {
          n72 = Format Into String(format string="Phasor Ratio: %#g\nAmplitude-averaged Lifetime: %#g ns\nIntensity-averaged Lifetime: %#g ns\n", error in=w228, w232, w230, w229) -> (resulting string=w233:string)  [unwired: 1 in, 1 out]
        }
      }
    }
  }
  n73 = Select(t="calibrated", s=w27, f="uncalibrated") -> (s? t:f=w21:string)
  n74 = node(w26) -> (w25:dbl)
  n75 = node(w39) -> (w38:dbl)
  n76 = node(w7) -> (w37:dbl)
  n77 = case shown="True" w13 {
    tunnel: [w245 w266] -> w45
    tunnel: w44 -> [w244 w265]
    tunnel: w43 -> [w243 w264]
    tunnel: [w242 w263] -> w42
    tunnel: w41 -> [w241 w262]
    tunnel: w40 -> [w240 w261]
    tunnel: w38 -> [w239 w248]
    tunnel: w37 -> [w238 w260]
    tunnel: w25 -> [w237 w250]
    tunnel: w14 -> [_ w256]
    tunnel: w9 -> [_ w257]
    tunnel: w7 -> [_ w255]
    tunnel: w21 -> [w235 w247]
    tunnel: w15 -> [w234 w246]
    frame False {
      # "no SDV"
      n78 = Format Into String(format string="Phasor added to plot %s f = %#g MHz:\n(g, s) = (%#g, %#g) [%s]\nPhase lifetime: %#g ns\nModulus lifetime: %#g ns\n%s" ("initial string"), error in=w244, w243, w238, w241, w240, w235, w239, w237, w234) -> (resulting string=w245:string, error out=w242:errorcluster)  [unwired: 1 in]
    }
    frame True {
      # "compute SDV"
      n79 = Unbundle By Name(w256) -> ("g"=w259:dbl, "s"=w258:dbl)
      n80 = call "Phasor Compute tau_phi SDV.vi"("Phasor Frequency"=w255, "Phasor SDV (g, s)"=w256, "Phasor (g, s)"=w257) -> ("tau_phi SDV"=w254:dbl[unit])  [unwired: 7 in, 1 out]
      n81 = call "Phasor Compute tau_m SDV.vi"("Phasor Frequency"=w255, "Phasor SDV (g, s)"=w256, "Phasor (g, s)"=w257) -> ("tau_m SDV"=w253:dbl[unit])  [unwired: 6 in, 2 out]
      n82 = node(w253) -> (w251:dbl)
      n83 = node(w254) -> (w249:dbl)
      n84 = Format Into String(format string="Phasor added to plot %s f = %#g MHz:\n(g, s) = (%#g +/- %#g, %#g +/- %#g) [%s]\nPhase lifetime: %#g +/- %#g ns\nModulus lifetime: %#g +/- %#g ns\n%s" ("initial string"), error in=w265, w264, w260, w262, w259, w261, w258, w247, w248, w249, w250, w251, w246) -> (resulting string=w266:string, error out=w263:errorcluster)  [unwired: 1 in]
    }
  }
  "Error Out" <- w42
  "Message" <- w45
